vi "Play Primary Sound.vi"(8 "error in (no error)":errorcluster, 11 "Ship in":refnum<class "Ship.lvclass">) -> (0 "error out":errorcluster)   [LabVIEW 2021, in "Ship.lvclass"]
uses:
  Ship.lvclass
  Ship.lvclass/Ship.ctl
  Resource Manager/Resource Manager.lvclass
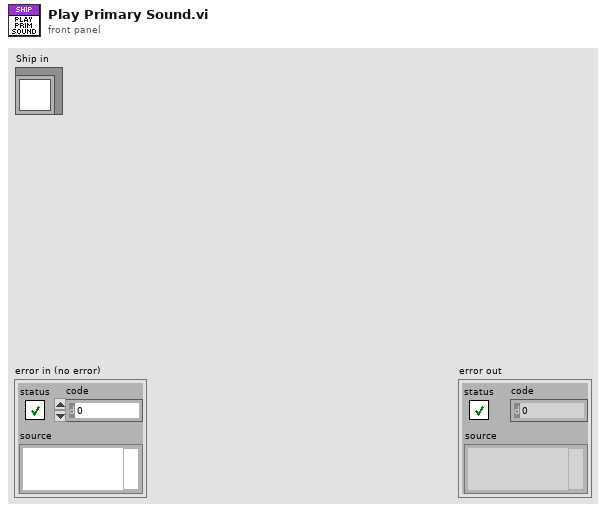
[diagram p1: front panel]
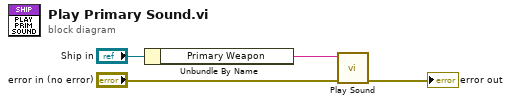
[diagram p0: block diagram]
diagram:
  n1 = Unbundle By Name("Ship in") -> ("Primary Weapon"=w3:string)
  n2 = call "Play Sound.vi"("error in (no error)"="error in (no error)", "Sound Name"=w3) -> ("error out"=→"error out":errorcluster)  [unwired: 9 in]
